vi "Test ADC.vi"(8 "error in (no error)":errorcluster, 11 "TestCase in":refnum<class "LecturaADC.lvclass">) -> (0 "error out":errorcluster, 3 "TestCase out":refnum<class "LecturaADC.lvclass">)   [LabVIEW 2020, in "LecturaADC.lvclass"]
uses:
  LecturaADC.lvclass
  Simulated Device/Simulated Device.lvclass
  <vilib>/addons/_JKI Toolkits/VI Tester/TestCase.llb/TestCase.lvclass
  C:/Program Files (x86)/National Instruments/LabVIEW 2020/vi.lib/addons/_JKI Toolkits/VI Tester/TestCase.llb/TestCase.lvclass
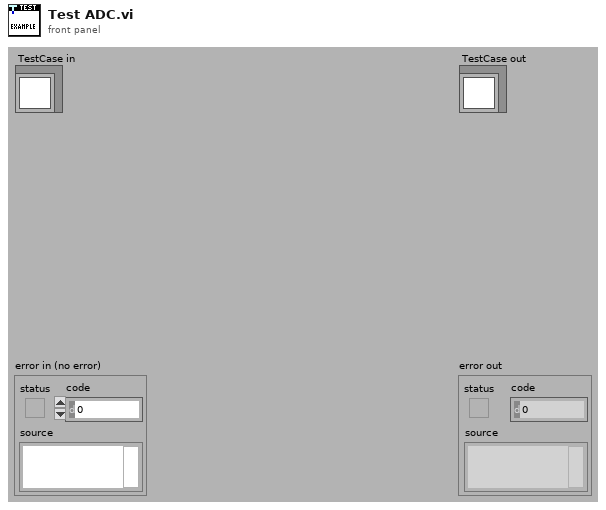
[diagram p1: front panel]
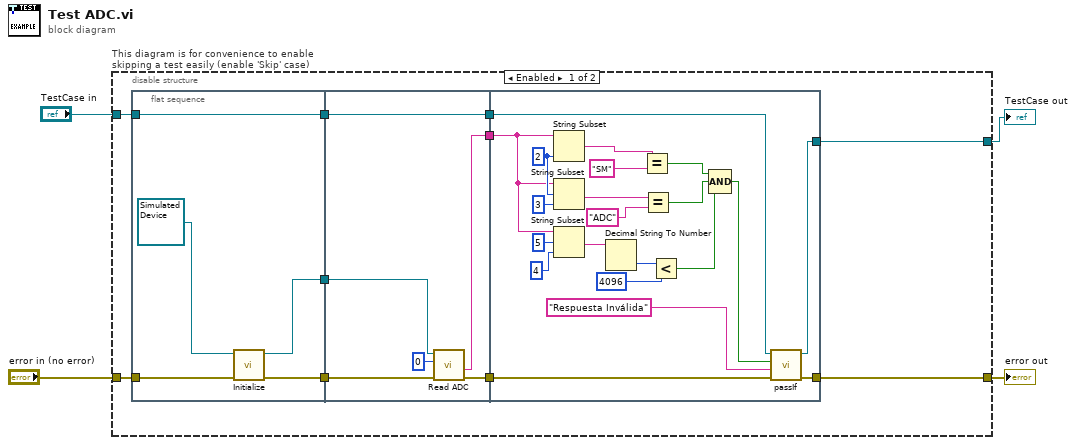
[diagram p0: block diagram]
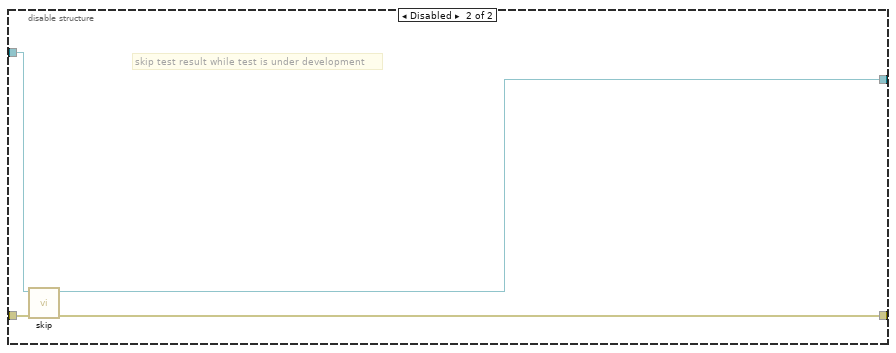
[diagram p2: hidden frame]
diagram:
  n1 = disable-structure "This diagram is for convenience to enable skipping a test easily (enable 'Skip' case)" shown="Enabled" {
    disable-tunnel: "TestCase in" -> [w14 w50]
    disable-tunnel: [w11 w48] -> w1
    disable-tunnel: [w12 w49] -> w3
    disable-tunnel: "error in (no error)" -> [w13 w47]
    frame Enabled {
      n2 = flat-sequence {
        tunnel: w14 -> [w19]
        tunnel: w13 -> [w17]
        tunnel: [w19] -> w10
        tunnel: [w16] -> w8
        tunnel: [w15] -> w6
        tunnel: w10 -> [w25]
        tunnel: [w25] -> w9
        tunnel: w8 -> [w24]
        tunnel: [w23] -> w7
        tunnel: w6 -> [w22]
        tunnel: [w20] -> w5
        tunnel: [w46] -> w12
        tunnel: [w45] -> w11
        tunnel: w9 -> [w44]
        tunnel: w7 -> [w43]
        tunnel: w5 -> [w40]
        frame #0 {
          n3 = call-dynamic "Initialize.vi"("error in (no error)"=w17, "Simulated Device in"=refnum<class "Simulated Device.lvclass"> refnum ("Simulated Device.lvclass")) -> ("error out"=w16:errorcluster, "Simulated Device out"=w15:refnum<class "Simulated Device.lvclass">)  [unwired: 7 in, 1 out]
        }
        frame #1 {
          n4 = call-dynamic "Read ADC.vi"("error in (no error)"=w24, "Channel"=u8 0, "Simulated Device in"=w22) -> ("error out"=w23:errorcluster, "Response"=w20:string)  [unwired: 5 in, 2 out]
        }
        frame #2 {
          w42 = 2 ("length (rest)")
          n5 = String Subset(string=w40, length (rest)=w42) -> (substring=w37:string)  [unwired: 1 in]
          n6 = String Subset(string=w40, offset (0)=w42, length (rest)=3 ("length (rest)")) -> (substring=w35:string)
          n7 = String Subset(string=w40, offset (0)=5, length (rest)=4 ("length (rest)")) -> (substring=w33:string)
          n8 = Decimal String To Number(string=w33) -> (number=w32:i32)  [unwired: 2 in, 1 out]
          n9 = Equal?(x=w37, y="SM") -> (x = y?=w30:bool)
          n10 = Equal?(x=w35, y="ADC") -> (x = y?=w29:bool)
          n11 = Less?(x=w32, y=4096) -> (x < y?=w28:bool)
          n12 = Compound Arithmetic op=AND(w30, w29, w28) -> (w27:bool)
          n13 = call-dynamic "passIf.vi"("error in (no error)"=w43, "message (\"\")"="Respuesta Inválida" ("message (\"\")"), "pass"=w27, "TestCase in"=w44) -> ("error out"=w46:errorcluster, "TestCase out"=w45:refnum<class "LecturaADC.lvclass">)  [unwired: 6 in]
        }
      }
    }
    frame Disabled {
      # "skip test result while test is under development"
      n14 = call <vilib>:"skip.vi"("error in (no error)"=w47, "TestCase in"=w50) -> ("error out"=w49:errorcluster, "TestCase out"=w48:refnum<class "LecturaADC.lvclass">)  [unwired: 8 in]
    }
  }
  "error out" <- w3
  "TestCase out" <- w1
